vi "Color(SubVI).vi"(0 "free":u32(colorbox) caption="Free", 1 "visObs":u32(colorbox) caption="Visible", 2 "start":u32(colorbox) caption="Start", 3 "goal":u32(colorbox) caption="Goal", 4 "invObs":u32(colorbox) caption="Invisible", 5 "path":u32(colorbox) caption="Path", 6 "uncertain":u32(colorbox) caption="Uncertain") -> (20 "freeCode":i32, 21 "visObsCode":i32, 22 "startCode":i32, 23 "goalCode":i32, 24 "invObsCode":i32, 25 "pathCode":i32, 26 "uncertainCode":i32, 27 "ZScale.MarkerVals[]":cluster{"cost":i32, "color":u32}[](array[cluster]))   [LabVIEW 2011]
doc: "Задает параметр цвета"
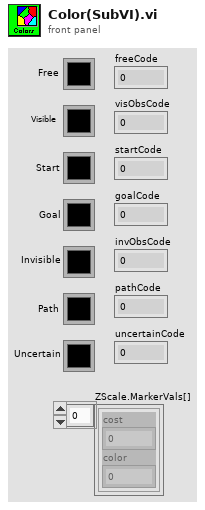
[diagram p1: front panel]
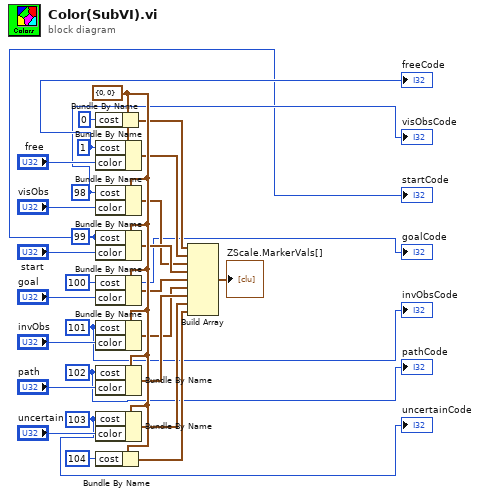
[diagram p0: block diagram]
diagram:
  w2 = 103 ("cost")
  w3 = 102 ("cost")
  w4 = 101 ("cost")
  w5 = 100 ("cost")
  w6 = 99 ("cost")
  w7 = 98 ("cost")
  w26 = cluster{"cost":i32, "color":u32} {"cost"=0, "color"=0} ("input cluster")
  w8 = 1
  n1 = Bundle By Name(cluster=w26, "cost"=0) -> (w24:cluster{"cost":i32, "color":u32})
  n2 = Bundle By Name(cluster=w26, "cost"=w8, "color"="free") -> (w23:cluster{"cost":i32, "color":u32})
  n3 = Bundle By Name(cluster=w26, "cost"=w7, "color"="visObs") -> (w17:cluster{"cost":i32, "color":u32})
  n4 = Bundle By Name(cluster=w26, "cost"=w6, "color"="start") -> (w18:cluster{"cost":i32, "color":u32})
  n5 = Bundle By Name(cluster=w26, "cost"=w5, "color"="goal") -> (w19:cluster{"cost":i32, "color":u32})
  n6 = Bundle By Name(cluster=w26, "cost"=w4, "color"="invObs") -> (w20:cluster{"cost":i32, "color":u32})
  n7 = Bundle By Name(cluster=w26, "cost"=w3, "color"="path") -> (w21:cluster{"cost":i32, "color":u32})
  n8 = Bundle By Name(cluster=w26, "cost"=w2, "color"="uncertain") -> (w25:cluster{"cost":i32, "color":u32})
  n9 = Bundle By Name(cluster=w26, "cost"=104) -> (w27:cluster{"cost":i32, "color":u32})
  n10 = Build Array(w24, w23, w17, w18, w19, w20, w21, w25, w27) -> (→"ZScale.MarkerVals[]":cluster{"cost":i32, "color":u32}[])
  "freeCode" <- w8
  "visObsCode" <- w7
  "startCode" <- w6
  "goalCode" <- w5
  "invObsCode" <- w4
  "pathCode" <- w3
  "uncertainCode" <- w2
